vi "ProcessDataFlowBlock_Parse.vi"(8 "error in (no error)":errorcluster, 11 "body":variant) -> (0 "error out":errorcluster, 3 "data":T1)   [LabVIEW 2017, in "DataFlow.lvlib"]
doc: "Converts the data set from the previous process in the Dataflow Script from variant data to its original cluster format."
uses:
  <vilib>/addons/InsightCM/Devices/Shared/Common/DataFlow/DataFlow.lvlib
  <vilib>/addons/InsightCM/Devices/Shared/Common/DataFlow/controls/Data.ctl
  <vilib>/addons/InsightCM/Utilities/DataAccessors/controls/wfmSGL_DVR.ctl
  <vilib>/addons/PointValueMap/controls/PointMap.ctl
  <vilib>/addons/InsightCM/Devices/Shared/Common/DataFlow/controls/Type.ctl
  <vilib>/addons/PointValueMap/PointValueMap.lvlib
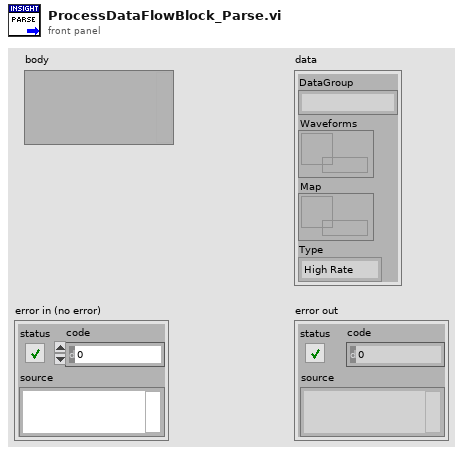
[diagram p1: front panel]
types:
  T1 = typedef "DataFlow.lvlib/Data.ctl" = cluster{"DataGroup":string, "Waveforms":T2, "Map":T3, "Type":T4}
  T2 = typedef "wfmSGL_DVR.ctl" = refnum<data-value>
  T3 = typedef "PointValueMap.lvlib/PointMap.ctl" = refnum<data-value>
  T4 = typedef "DataFlow.lvlib/Type.ctl" = enum16{"High Rate", "Low Rate", "Burst Mode"}
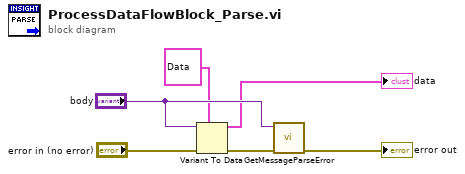
[diagram p0: block diagram]
diagram:
  n1 = Variant To Data(error in="error in (no error)", type=T1 {"DataGroup"="", "Waveforms"=refnum, "Map"=refnum, "Type"=enum."High Rate"} ("data"), Variant="body") -> (data=→"data":T1, error out=w6:errorcluster)
  n2 = call <vilib>:"GetMessageParseError.vi"("error in (no error)"=w6, "body"="body") -> ("error out"=→"error out":errorcluster)  [unwired: 7 in, 2 out]
